vi "Check if FP Already Open.vi"(8 "error in":errorcluster, 11 "Flex Dialog in":refnum<class "Flex UI Dialog.lvclass">) -> (0 "error out":errorcluster, 3 "Flex Dialog out":refnum<class "Flex UI Dialog.lvclass">)   [LabVIEW 2016, in "Flex UI Dialog.lvclass"]
doc: "Determines if the front panel was already open and stores the result in a boolean flag."
uses:
  Flex UI Dialog.lvclass
  C:/VI Packages/Flex UI/Flex UI (Parent)/Flex UI.lvclass
  Flex UI (Parent)/Flex UI.lvclass/Flex UI.ctl
  Flex UI Dialog.lvclass/Flex UI Dialog.ctl
  Flex UI (Parent)/Flex UI.lvclass
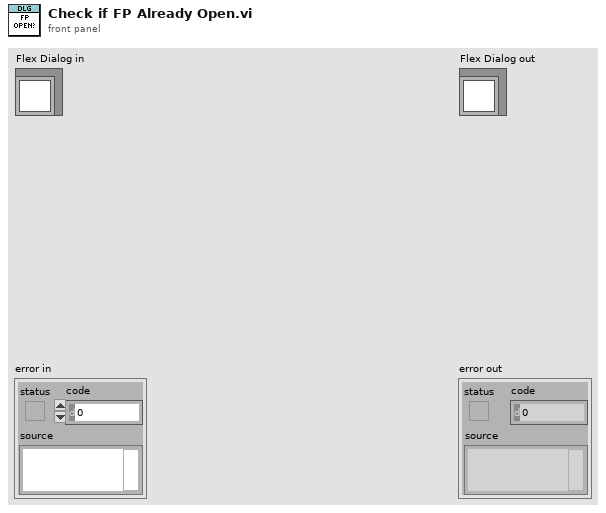
[diagram p1: front panel]
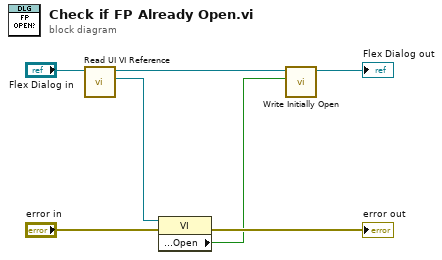
[diagram p0: block diagram]
diagram:
  n1 = call "Read UI VI Reference.vi"("Flex UI in"="Flex Dialog in") -> ("UI VI Reference"=w3:refnum<vi>, "Flex UI out"=w4:refnum<class "Flex UI Dialog.lvclass">)  [unwired: 9 in]
  n2 = property class="VI"(reference=w3, error in="error in") -> (error out=→"error out":errorcluster, "Front Panel.Open"=w1:bool)  [unwired: 1 out]
  n3 = call "Write Initially Open.vi"("Initially Open?"=w1, "Flex Dialog in"=w4) -> ("Flex Dialog out"=→"Flex Dialog out":refnum<class "Flex UI Dialog.lvclass">)  [unwired: 9 in]
